vi "Ignore Hidden Files.vi"(8 "error in (no error)":errorcluster, 11 "Paths":path[](array[path])) -> (0 "error out":errorcluster, 3 "Paths out":path[](array[path]))   [LabVIEW 2016]
doc: "Given a list of files, <b>Paths</b>, returns a list with hidden files removed."
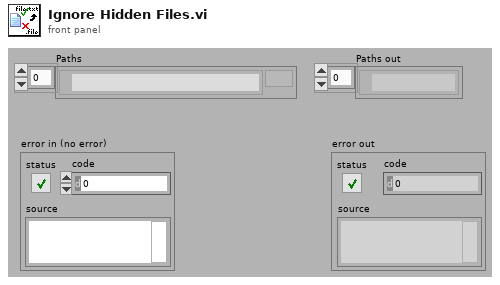
[diagram p1: front panel]
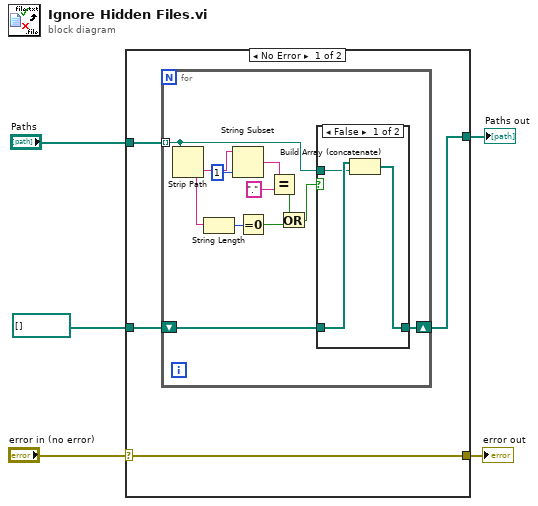
[diagram p0: block diagram]
diagram:
  n1 = case shown="No Error" "error in (no error)" {
    selector: "error in (no error)" -> [w6 w26]
    tunnel: path[] [] ("file names") -> [w8 _]
    tunnel: [w7 w25] -> w4
    tunnel: [w6 w26] -> w2
    tunnel: "Paths" -> [w9 w25]
    frame No Error {
      n2 = for {
        tunnel: w9 -> [w15] mode=indexing
        shift-right: [w17] -> w7
        shift-left: w8 -> [w16]
        n3 = Strip Path(path=w15) -> (name=w13:string)  [unwired: 1 out]
        n4 = String Length(string=w13) -> (length=w12:i32)
        n5 = String Subset(string=w13, length (rest)=1 ("length (rest)")) -> (substring=w18:string)  [unwired: 1 in]
        n6 = Equal To 0?(x=w12) -> (x = 0?=w11:bool)
        n7 = Equal?(x=w18, y=".") -> (x = y?=w10:bool)
        n8 = Or(x=w10, y=w11) -> (x .or. y?=w14:bool)
        n9 = case shown="False" w14 {
          tunnel: [w23 w24] -> w17
          tunnel: w16 -> [w22 w24]
          tunnel: w15 -> [w21 _]
          frame False {
            n10 = Build Array (concatenate)(w22, w21) -> (w23:path[])
          }
          frame True {
          }
        }
      }
    }
    frame Error {
    }
  }
  "Paths out" <- w4
  "error out" <- w2
